vi "openbci_is_daisy.vi"(11 "reset_str_in":string) -> (3 "daisy board?":bool)   [LabVIEW 2013]
doc: "Reads Transmission until EOT (EOT) is found"
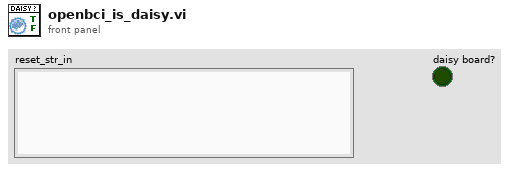
[diagram p1: front panel]
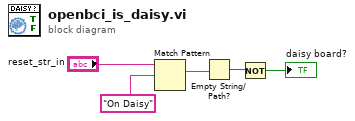
[diagram p0: block diagram]
diagram:
  n1 = Match Pattern(string="reset_str_in", regular expression="On Daisy" ("true string")) -> (match substring=w3:string)  [unwired: 1 in, 3 out]
  n2 = Empty String/Path?(string/path=w3) -> (empty?=w2:bool)
  n3 = Not(x=w2) -> (.not. x?=→"daisy board?":bool)
